vi "Write to System Log.vi"(8 "error in (no error)":errorcluster, 11 "Message":string) -> (0 "error out":errorcluster)   [LabVIEW 2018, in "File IO.lvlib"]
doc: "This subVI enqueues the named action in to the communications queue along with the input data."
uses:
  File IO.lvlib
  Private Controls/Module Data.ctl
  Private Controls/Module Action.ctl
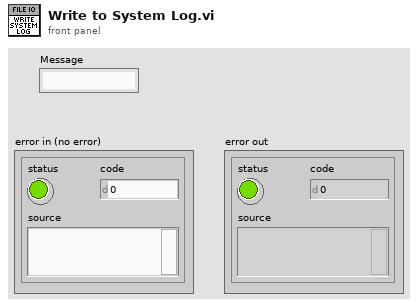
[diagram p1: front panel]
types:
  T1 = typedef "File IO.lvlib/Module Action.ctl" = enum8{"Timeout", "OpenReport", "Continue Test", "Init", "Error", "Exit", "Save Accel Data", "Set Recording State", "Log APU RunTime", "Start New Test", "Create New Reports", "Write to System Log", "Save Variables", "Load APU Setup File", "Increment Run Count", "Write To Report"}
  T2 = typedef "File IO.lvlib/Module Data.ctl" = cluster{"Data":variant, "Action":T1}
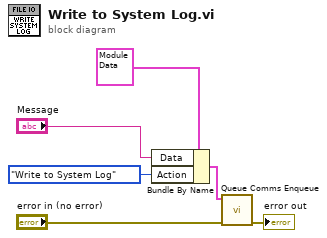
[diagram p0: block diagram]
diagram:
  n1 = Bundle By Name(cluster=T2 {"Data"=variant, "Action"=enum."Init"} ("element"), "Data"="Message", "Action"=Module_Action."Write to System Log") -> (w5:T2)
  n2 = call "Queue Comms Enqueue.vi"("error in (no error)"="error in (no error)", "element"=w5) -> ("error out"=→"error out":errorcluster)  [unwired: 9 in]
